vi "Read Channel Names.vi"(8 "error in (no error)":errorcluster, 11 "Logging Data in":refnum<class "Logging Data.lvclass">) -> (0 "error out":errorcluster, 2 "Channel Names":string[](array[string]), 3 "Logging Data out":refnum<class "Logging Data.lvclass">)   [LabVIEW 2024, in "Logging Data.lvlib" / "Logging Data.lvclass"]
uses:
  Logging Data.lvclass
  Logging Data.lvclass/Logging Data.ctl
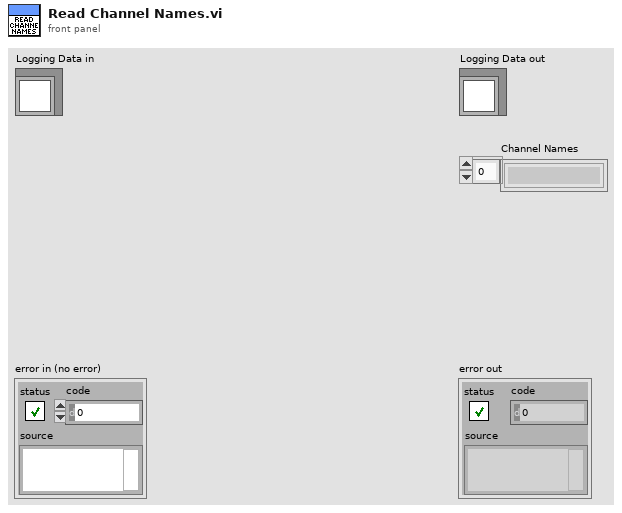
[diagram p1: front panel]
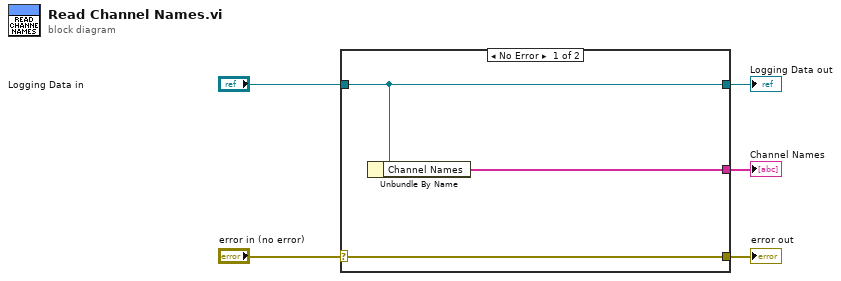
[diagram p0: block diagram]
diagram:
  n1 = case shown="No Error" "error in (no error)" {
    selector: "error in (no error)" -> [w8 w9]
    tunnel: [w8 w9] -> w4
    tunnel: [w7 w10] -> w2
    tunnel: "Logging Data in" -> [w7 w10]
    tunnel: [w6 _] -> w1
    frame No Error {
      n2 = Unbundle By Name(w7) -> ("Channel Names"=w6:string[])
    }
    frame Error {
    }
  }
  "error out" <- w4
  "Logging Data out" <- w2
  "Channel Names" <- w1
